vi "ICM Load Channel Scaling Config.vi"(8 "error in (no error)":errorcluster, 11 "Scalings":T1[](array[typedef])) -> (0 "error out":errorcluster, 1 "Scaling Classes":refnum<class "Scaling.lvclass">[](array[class]), 2 "Used Scalings":string[](array[string]), 3 "Scalings Out":T1[](array[typedef]))   [LabVIEW 2024]
doc: "ICM Load Channel Scaling Config.vi\n\nThis VI takes the channel scalings found with the ICM Read Channel Scalings.vi and assembles an array of the class references for all the Scaling child classes needed to execute the scalings. Assembling this array when the program is initialized prevents the child scaling classes from having to access their configuration on disk when scalings are executed.\n\nInstrument Communication Module Version 1.0\nDecember, 2017 Original Code Consulting David Thomson\n www.originalcode.com"
uses:
  Scaling/Scaling Def.ctl
  Scaling/Scaling.lvclass
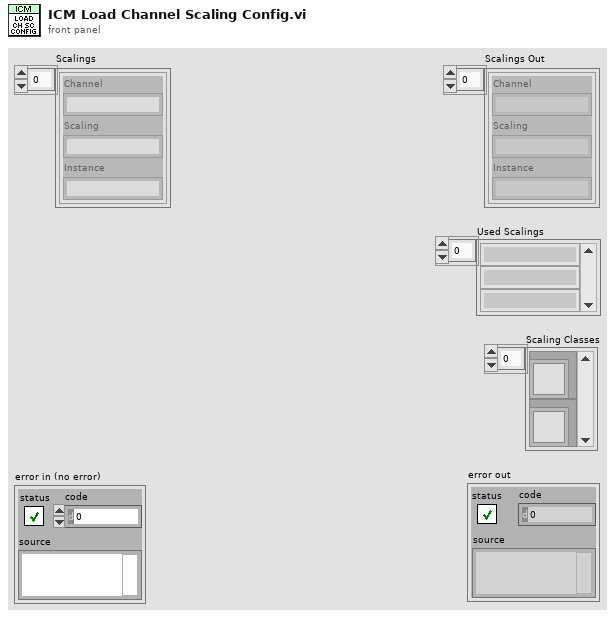
[diagram p1: front panel]
types:
  T1 = typedef "Scaling Def.ctl" = cluster{"Channel":string, "Scaling":string, "Instance":string}
  T2 = enum32{"invalid app kind", "Development System", "Run Time System", "Student Edition", "Embedded LabVIEW", "Evaluation", "Custom"}
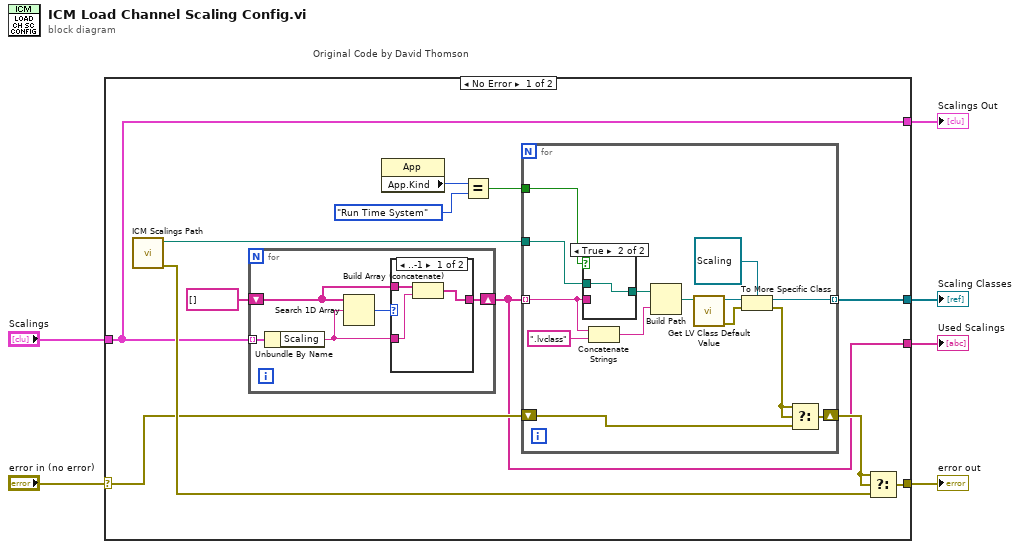
[diagram p0: block diagram]
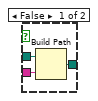
[diagram p2: hidden frame]
diagram:
  n1 = case "Original Code by David Thomson" shown="No Error" "error in (no error)" {
    selector: "error in (no error)" -> [w15 w47]
    tunnel: [w16 w47] -> w5
    tunnel: "Scalings" -> [w10 w46]
    tunnel: [w12 _] -> w3
    tunnel: [w11 _] -> w2
    tunnel: [w10 w46] -> w1
    frame No Error {
      n2 = call "ICM Scalings Path.vi"() -> ("error out"=w18:errorcluster, "ICM Scalings Path"=w17:path)  [unwired: 10 in]
      n3 = for {
        tunnel: w10 -> [w41] mode=indexing
        shift-right: [w39] -> w12
        shift-left: string[] [] -> [w38]
        n4 = Unbundle By Name(w41) -> ("Scaling"=w37:string)
        n5 = Search 1D Array(1D array=w38, element=w37) -> (index of element=w40:i32)  [unwired: 1 in]
        n6 = case shown="..-1" w40 {
          tunnel: [w42 w45] -> w39
          tunnel: w38 -> [w44 w45]
          tunnel: w37 -> [w43 _]
          frame ..-1 {
            n7 = Build Array (concatenate)(w44, w43) -> (w42:string[])
          }
          frame 0.. {
          }
        }
      }
      n8 = property class="App"() -> ("App.Kind"=w9:T2)  [unwired: 2 in, 2 out]
      n9 = Equal?(x=w9, y=T2."Run Time System" ("Application:Kind")) -> (x = y?=w7:bool)
      n10 = for {
        tunnel: w12 -> [w20] mode=indexing
        tunnel: [w25] -> w11 mode=indexing
        shift-right: [w23] -> w13
        shift-left: w15 -> [w22]
        tunnel: w17 -> [w21]
        tunnel: w7 -> [w19]
        n11 = case shown="True" w19 {
          tunnel: [w35 w36] -> w26
          tunnel: w21 -> [w34 w36]
          tunnel: w20 -> [w33 _]
          frame False {
            n12 = Build Path(base path=w34, name or relative path=w33) -> (appended path=w35:path)
          }
          frame True {
          }
        }
        n13 = Concatenate Strings(w20, ".lvclass" ("string")) -> (w32:string)
        n14 = Build Path(base path=w26, name or relative path=w32) -> (appended path=w30:path)
        n15 = call <vilib>:"Get LV Class Default Value.vi"("class path"=w30) -> ("error out"=w27:errorcluster, "object"=w29:refnum<class>)  [unwired: 9 in]
        n16 = To More Specific Class(target class=refnum<class "Scaling.lvclass"> refnum ("Scaling.lvclass"), reference=w29, error in=w27) -> (specific class reference=w25:refnum<class "Scaling.lvclass">, error out=w24:errorcluster)
        n17 = Select(t=w24, s=w24, f=w22) -> (s? t:f=w23:errorcluster)
      }
      n18 = Select(t=w13, s=w13, f=w18) -> (s? t:f=w16:errorcluster)
    }
    frame Error {
    }
  }
  "error out" <- w5
  "Used Scalings" <- w3
  "Scaling Classes" <- w2
  "Scalings Out" <- w1
